vi "SpinAuxs.vi"(4 "error in":errorcluster, 6 "Init":bool, 7 "IntakeSpeed":dbl, 8 "Time":dbl, 9 "BeltSpeed":dbl, 10 "FeederSpeed":dbl, 11 "ShootSpeed":dbl) -> (1 "error out":errorcluster, 3 "Finished":bool)   [LabVIEW 2020]
uses:
  AuxGlobals.vi
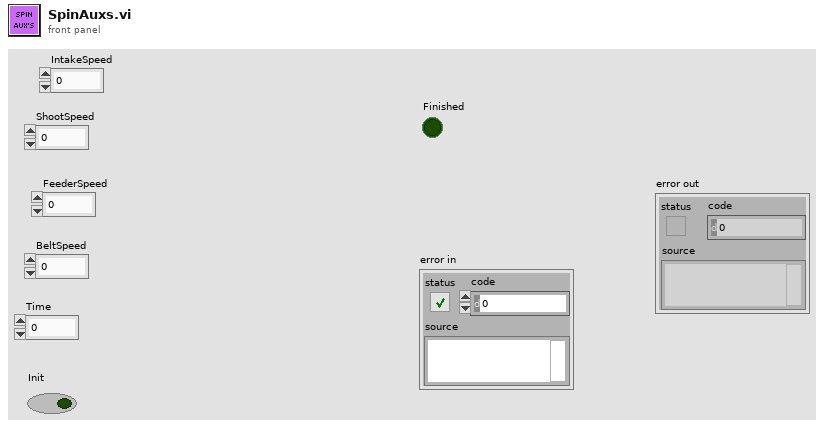
[diagram p1: front panel]
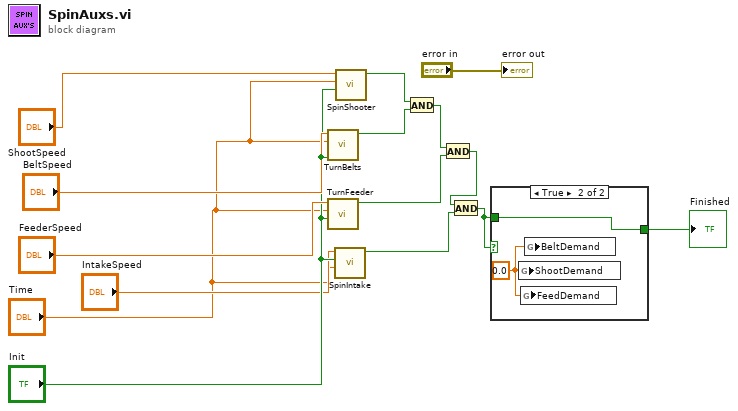
[diagram p0: block diagram]
diagram:
  n1 = call "TurnBelts.vi"("Initation?"="Init", "Time"="Time", "BeltSpeed"="BeltSpeed") -> ("Finished"=w10:bool)  [unwired: 7 in, 1 out]
  n2 = call "TurnFeeder.vi"("Initation?"="Init", "Time"="Time", "Speed"="FeederSpeed") -> ("Finished"=w12:bool)  [unwired: 7 in, 1 out]
  n3 = call "SpinIntake.vi"("Time"="Time", "Initation?"="Init", "Speed"="IntakeSpeed") -> ("Finished"=w2:bool)  [unwired: 7 in, 1 out]
  n4 = call "SpinShooter.vi"("Initation?"="Init", "Time"="Time", "Speed"="ShootSpeed") -> ("Finished"=w9:bool)  [unwired: 7 in, 1 out]
  n5 = And(x=w9, y=w10) -> (x .and. y?=w11:bool)
  n6 = And(x=w11, y=w12) -> (x .and. y?=w3:bool)
  n7 = And(x=w3, y=w2) -> (x .and. y?=w1:bool)
  n8 = case shown="True" w1 {
    tunnel: [w16 w18] -> w8
    tunnel: w1 -> [w16 w18]
    frame False {
    }
    frame True {
      w17 = 0.0 ("ShootDemand")
      n9 = global write "AuxGlobals.vi" "ShootDemand"(w17) -> ()
      n10 = global write "AuxGlobals.vi" "FeedDemand"(w17) -> ()
      n11 = global write "AuxGlobals.vi" "BeltDemand"(w17) -> ()
    }
  }
  "Finished" <- w8
  "error out" <- "error in"
